vi "Yellow Place.vi"   [LabVIEW 2019]
uses:
  Global Var.vi
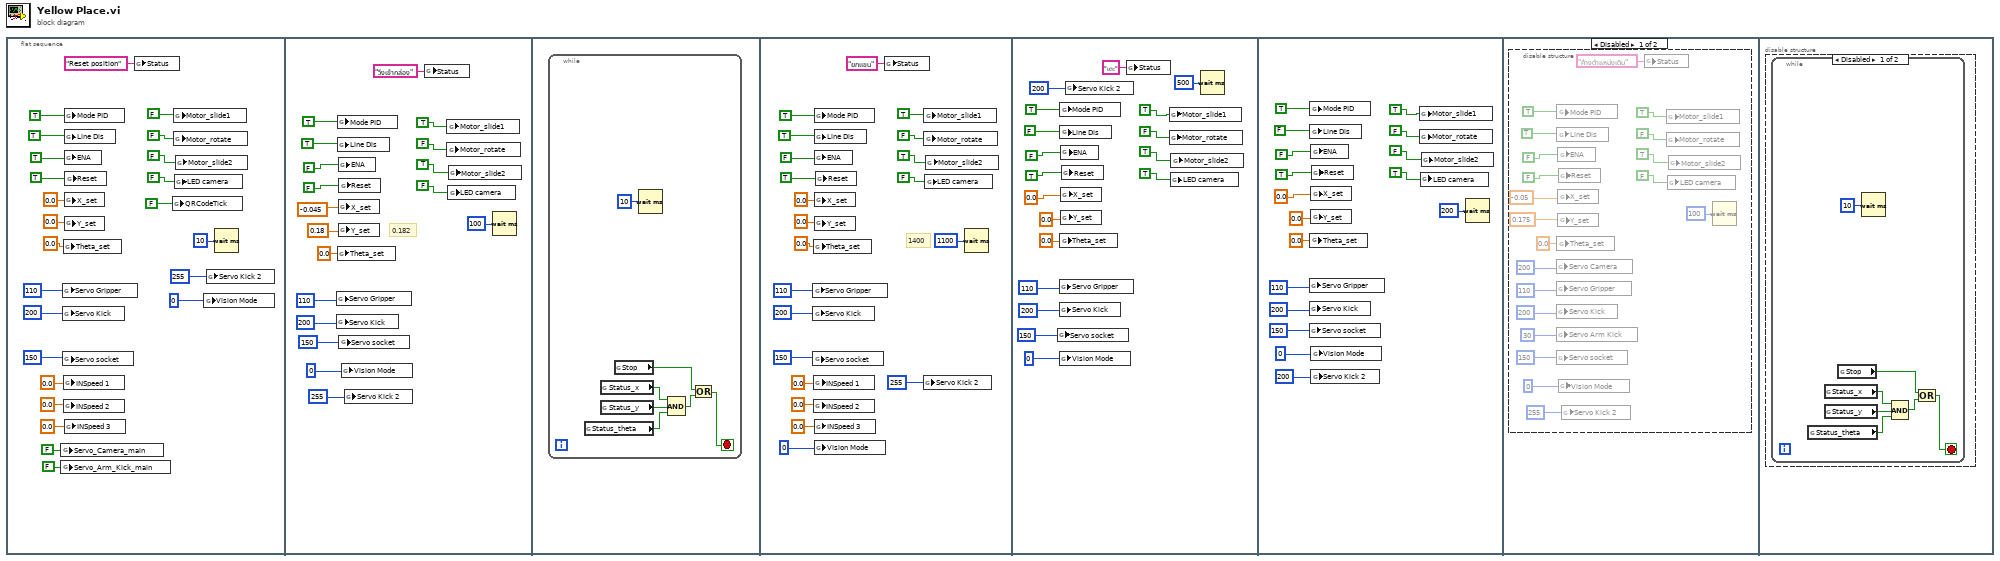
[diagram p0: block diagram]
diagram:
  n1 = flat-sequence {
    frame #0 {
      n2 = global write "Global Var.vi" "Servo_Camera_main"(FALSE ("Mode PID")) -> ()
      n3 = global write "Global Var.vi" "Servo_Arm_Kick_main"(FALSE ("Mode PID")) -> ()
      n4 = global write "Global Var.vi" "Servo Gripper"(u8 110 ("Servo Camera")) -> ()
      n5 = global write "Global Var.vi" "Servo Kick"(u8 200 ("Servo Camera")) -> ()
      n6 = global write "Global Var.vi" "Servo socket"(u8 150 ("Servo Camera")) -> ()
      n7 = global write "Global Var.vi" "Theta_set"(0.0 ("Theta_set")) -> ()
      n8 = global write "Global Var.vi" "INSpeed 1"(0.0 ("X_set")) -> ()
      n9 = global write "Global Var.vi" "INSpeed 2"(0.0 ("Y_set")) -> ()
      n10 = global write "Global Var.vi" "Mode PID"(TRUE ("Mode PID")) -> ()
      n11 = global write "Global Var.vi" "Line Dis"(TRUE ("Mode PID")) -> ()
      n12 = global write "Global Var.vi" "ENA"(TRUE ("ENA")) -> ()
      n13 = global write "Global Var.vi" "X_set"(0.0 ("X_set")) -> ()
      n14 = global write "Global Var.vi" "Y_set"(0.0 ("Y_set")) -> ()
      n15 = global write "Global Var.vi" "INSpeed 3"(0.0 ("Theta_set")) -> ()
      n16 = global write "Global Var.vi" "Reset"(TRUE ("ENA")) -> ()
      n17 = global write "Global Var.vi" "Status"("Reset position" ("Status")) -> ()
      n18 = global write "Global Var.vi" "QRCodeTick"(FALSE ("Mode PID")) -> ()
      n19 = global write "Global Var.vi" "Motor_slide1"(FALSE ("Mode PID")) -> ()
      n20 = global write "Global Var.vi" "Motor_rotate"(FALSE ("ENA")) -> ()
      n21 = global write "Global Var.vi" "LED camera"(FALSE ("LED camera")) -> ()
      n22 = global write "Global Var.vi" "Motor_slide2"(FALSE ("ENA")) -> ()
      n23 = global write "Global Var.vi" "Vision Mode"(i16 0 ("Vision Mode")) -> ()
      n24 = global write "Global Var.vi" "Servo Kick 2"(u8 255 ("Servo Camera")) -> ()
      n25 = Wait (ms)(milliseconds to wait=u32 10) -> ()  [unwired: 1 out]
    }
    frame #1 {
      # "0.182"
      n26 = global write "Global Var.vi" "Servo Gripper"(u8 110 ("Servo Camera")) -> ()
      n27 = global write "Global Var.vi" "Servo Kick"(u8 200 ("Servo Camera")) -> ()
      n28 = global write "Global Var.vi" "Mode PID"(TRUE ("Mode PID")) -> ()
      n29 = global write "Global Var.vi" "Line Dis"(TRUE ("Mode PID")) -> ()
      n30 = global write "Global Var.vi" "Theta_set"(0.0 ("Theta_set")) -> ()
      n31 = global write "Global Var.vi" "ENA"(FALSE ("ENA")) -> ()
      n32 = global write "Global Var.vi" "X_set"(-0.045 ("X_set")) -> ()
      n33 = global write "Global Var.vi" "Y_set"(0.18 ("Y_set")) -> ()
      n34 = global write "Global Var.vi" "Reset"(FALSE ("ENA")) -> ()
      n35 = global write "Global Var.vi" "Servo socket"(u8 150 ("Servo Camera")) -> ()
      n36 = global write "Global Var.vi" "Vision Mode"(i16 0 ("Vision Mode")) -> ()
      n37 = global write "Global Var.vi" "Servo Kick 2"(u8 255 ("Servo Camera")) -> ()
      n38 = global write "Global Var.vi" "Status"("วิ่งเข้ากล่อง" ("Status")) -> ()
      n39 = global write "Global Var.vi" "Motor_slide1"(TRUE ("Mode PID")) -> ()
      n40 = global write "Global Var.vi" "Motor_rotate"(FALSE ("ENA")) -> ()
      n41 = global write "Global Var.vi" "LED camera"(FALSE ("LED camera")) -> ()
      n42 = global write "Global Var.vi" "Motor_slide2"(TRUE ("ENA")) -> ()
      n43 = Wait (ms)(milliseconds to wait=u32 100) -> ()  [unwired: 1 out]
    }
    frame #2 {
      n44 = while {
        stop <- w45 stop-if-true
        n45 = global read "Global Var.vi" "Status_theta"() -> (w47:bool)
        n46 = global read "Global Var.vi" "Status_x"() -> (w48:bool)
        n47 = global read "Global Var.vi" "Status_y"() -> (w49:bool)
        n48 = global read "Global Var.vi" "Stop"() -> (w43:bool)
        n49 = Wait (ms)(milliseconds to wait=u32 10) -> ()  [unwired: 1 out]
        n50 = Compound Arithmetic op=AND(w48, w49, w47) -> (w44:bool)
        n51 = Or(x=w43, y=w44) -> (x .or. y?=w45:bool)
      }
    }
    frame #3 {
      # "1400"
      n52 = global write "Global Var.vi" "Servo Gripper"(u8 110 ("Servo Camera")) -> ()
      n53 = global write "Global Var.vi" "Servo Kick"(u8 200 ("Servo Camera")) -> ()
      n54 = global write "Global Var.vi" "Servo socket"(u8 150 ("Servo Camera")) -> ()
      n55 = global write "Global Var.vi" "Theta_set"(0.0 ("Theta_set")) -> ()
      n56 = global write "Global Var.vi" "INSpeed 1"(0.0 ("X_set")) -> ()
      n57 = global write "Global Var.vi" "INSpeed 2"(0.0 ("Y_set")) -> ()
      n58 = global write "Global Var.vi" "Mode PID"(TRUE ("Mode PID")) -> ()
      n59 = global write "Global Var.vi" "Line Dis"(TRUE ("Mode PID")) -> ()
      n60 = global write "Global Var.vi" "ENA"(FALSE ("ENA")) -> ()
      n61 = global write "Global Var.vi" "X_set"(0.0 ("X_set")) -> ()
      n62 = global write "Global Var.vi" "Y_set"(0.0 ("Y_set")) -> ()
      n63 = global write "Global Var.vi" "INSpeed 3"(0.0 ("Theta_set")) -> ()
      n64 = global write "Global Var.vi" "Vision Mode"(i16 0 ("Vision Mode")) -> ()
      n65 = global write "Global Var.vi" "Reset"(TRUE ("ENA")) -> ()
      n66 = global write "Global Var.vi" "Status"("ยกเเขน" ("Status")) -> ()
      n67 = global write "Global Var.vi" "Servo Kick 2"(u8 255 ("Servo Camera")) -> ()
      n68 = global write "Global Var.vi" "Motor_slide1"(TRUE ("Mode PID")) -> ()
      n69 = global write "Global Var.vi" "Motor_rotate"(FALSE ("ENA")) -> ()
      n70 = global write "Global Var.vi" "LED camera"(FALSE ("LED camera")) -> ()
      n71 = global write "Global Var.vi" "Motor_slide2"(TRUE ("ENA")) -> ()
      n72 = Wait (ms)(milliseconds to wait=u32 1100) -> ()  [unwired: 1 out]
    }
    frame #4 {
      n73 = global write "Global Var.vi" "Servo socket"(u8 150 ("Servo Camera")) -> ()
      n74 = global write "Global Var.vi" "Servo Gripper"(u8 110 ("Servo Camera")) -> ()
      n75 = global write "Global Var.vi" "Servo Kick"(u8 200 ("Servo Camera")) -> ()
      n76 = global write "Global Var.vi" "Vision Mode"(i16 0 ("Vision Mode")) -> ()
      n77 = global write "Global Var.vi" "Mode PID"(TRUE ("Mode PID")) -> ()
      n78 = global write "Global Var.vi" "Line Dis"(FALSE ("Mode PID")) -> ()
      n79 = global write "Global Var.vi" "Theta_set"(0.0 ("Theta_set")) -> ()
      n80 = global write "Global Var.vi" "ENA"(FALSE ("ENA")) -> ()
      n81 = global write "Global Var.vi" "X_set"(0.0 ("X_set")) -> ()
      n82 = global write "Global Var.vi" "Y_set"(0.0 ("Y_set")) -> ()
      n83 = global write "Global Var.vi" "Reset"(TRUE ("ENA")) -> ()
      n84 = global write "Global Var.vi" "Servo Kick 2"(u8 200 ("Servo Camera")) -> ()
      n85 = global write "Global Var.vi" "Status"("เตะ" ("Status")) -> ()
      n86 = global write "Global Var.vi" "Motor_slide1"(TRUE ("Mode PID")) -> ()
      n87 = global write "Global Var.vi" "Motor_rotate"(FALSE ("ENA")) -> ()
      n88 = global write "Global Var.vi" "LED camera"(TRUE ("LED camera")) -> ()
      n89 = global write "Global Var.vi" "Motor_slide2"(TRUE ("ENA")) -> ()
      n90 = Wait (ms)(milliseconds to wait=u32 500) -> ()  [unwired: 1 out]
    }
    frame #5 {
      n91 = global write "Global Var.vi" "Servo Gripper"(u8 110 ("Servo Camera")) -> ()
      n92 = global write "Global Var.vi" "Servo Kick"(u8 200 ("Servo Camera")) -> ()
      n93 = global write "Global Var.vi" "Servo socket"(u8 150 ("Servo Camera")) -> ()
      n94 = global write "Global Var.vi" "Mode PID"(TRUE ("Mode PID")) -> ()
      n95 = global write "Global Var.vi" "Line Dis"(FALSE ("Mode PID")) -> ()
      n96 = global write "Global Var.vi" "Theta_set"(0.0 ("Theta_set")) -> ()
      n97 = global write "Global Var.vi" "ENA"(FALSE ("ENA")) -> ()
      n98 = global write "Global Var.vi" "X_set"(0.0 ("X_set")) -> ()
      n99 = global write "Global Var.vi" "Y_set"(0.0 ("Y_set")) -> ()
      n100 = global write "Global Var.vi" "Vision Mode"(i16 0 ("Vision Mode")) -> ()
      n101 = global write "Global Var.vi" "Servo Kick 2"(u8 200 ("Servo Camera")) -> ()
      n102 = global write "Global Var.vi" "Reset"(TRUE ("ENA")) -> ()
      n103 = global write "Global Var.vi" "Motor_slide1"(TRUE ("Mode PID")) -> ()
      n104 = global write "Global Var.vi" "Motor_rotate"(FALSE ("ENA")) -> ()
      n105 = global write "Global Var.vi" "LED camera"(TRUE ("LED camera")) -> ()
      n106 = global write "Global Var.vi" "Motor_slide2"(FALSE ("ENA")) -> ()
      n107 = Wait (ms)(milliseconds to wait=u32 200) -> ()  [unwired: 1 out]
    }
    frame #6 {
      n108 = disable-structure shown="Disabled" {
        frame Disabled {
          n109 = global write "Global Var.vi" "Servo Camera"(u8 200 ("Servo Camera")) -> ()
          n110 = global write "Global Var.vi" "Servo Gripper"(u8 110 ("Servo Camera")) -> ()
          n111 = global write "Global Var.vi" "Servo Kick"(u8 200 ("Servo Camera")) -> ()
          n112 = global write "Global Var.vi" "Servo Arm Kick"(u8 30 ("Servo Camera")) -> ()
          n113 = global write "Global Var.vi" "Servo socket"(u8 150 ("Servo Camera")) -> ()
          n114 = global write "Global Var.vi" "Mode PID"(TRUE ("Mode PID")) -> ()
          n115 = global write "Global Var.vi" "Line Dis"(TRUE ("Mode PID")) -> ()
          n116 = global write "Global Var.vi" "Theta_set"(0.0 ("Theta_set")) -> ()
          n117 = global write "Global Var.vi" "ENA"(FALSE ("ENA")) -> ()
          n118 = global write "Global Var.vi" "X_set"(-0.05 ("X_set")) -> ()
          n119 = global write "Global Var.vi" "Y_set"(0.175 ("Y_set")) -> ()
          n120 = global write "Global Var.vi" "Reset"(FALSE ("ENA")) -> ()
          n121 = global write "Global Var.vi" "Vision Mode"(i16 0 ("Vision Mode")) -> ()
          n122 = global write "Global Var.vi" "Servo Kick 2"(u8 255 ("Servo Camera")) -> ()
          n123 = global write "Global Var.vi" "Status"("ค้างต่ำแหน่งเดิม" ("Status")) -> ()
          n124 = global write "Global Var.vi" "Motor_slide1"(TRUE ("Mode PID")) -> ()
          n125 = global write "Global Var.vi" "Motor_rotate"(FALSE ("ENA")) -> ()
          n126 = global write "Global Var.vi" "LED camera"(FALSE ("LED camera")) -> ()
          n127 = global write "Global Var.vi" "Motor_slide2"(TRUE ("ENA")) -> ()
          n128 = Wait (ms)(milliseconds to wait=u32 100) -> ()  [unwired: 1 out]
        }
        frame Enabled {
        }
      }
    }
    frame #7 {
      n129 = disable-structure shown="Disabled" {
        frame Disabled {
          n130 = while {
            stop <- w128 stop-if-true
            n131 = global read "Global Var.vi" "Status_theta"() -> (w130:bool)
            n132 = global read "Global Var.vi" "Status_x"() -> (w131:bool)
            n133 = global read "Global Var.vi" "Status_y"() -> (w132:bool)
            n134 = global read "Global Var.vi" "Stop"() -> (w126:bool)
            n135 = Wait (ms)(milliseconds to wait=u32 10) -> ()  [unwired: 1 out]
            n136 = Compound Arithmetic op=AND(w131, w132, w130) -> (w127:bool)
            n137 = Or(x=w126, y=w127) -> (x .or. y?=w128:bool)
          }
        }
        frame Enabled {
        }
      }
    }
  }
